vi "Write Value.vi"(8 "error in (no error)":errorcluster, 10 "Value":i32, 11 "sfixed32 in":refnum<class "sfixed32.lvclass">) -> (0 "error out":errorcluster, 3 "sfixed32 out":refnum<class "sfixed32.lvclass">)   [LabVIEW 2020, in "Protobuf RAW.lvlib" / "sfixed32.lvclass"]
uses:
  sfixed32.lvclass
  sfixed32.lvclass/sfixed32.ctl
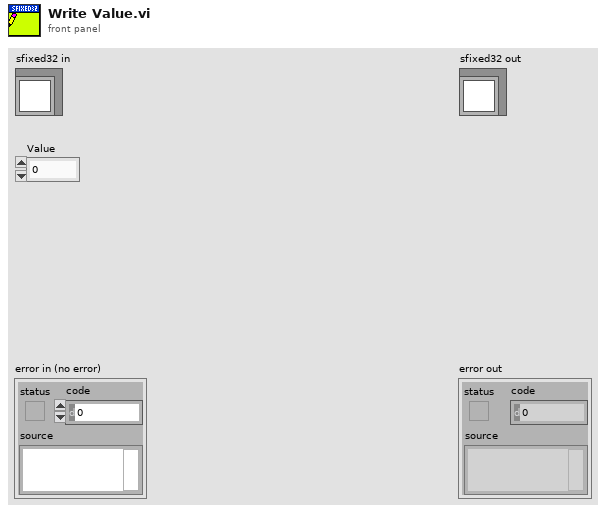
[diagram p1: front panel]
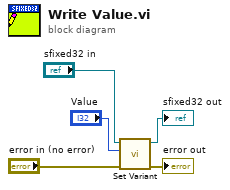
[diagram p0: block diagram]
diagram:
  n1 = call-dynamic "Set Variant.vi"("error in (no error)"="error in (no error)", "Value"="Value", "Proto Type Common in"="sfixed32 in") -> ("error out"=→"error out":errorcluster, "Proto Type Common out"=→"sfixed32 out":refnum<class "sfixed32.lvclass">)  [unwired: 7 in]
